vi "init_DAC_do_chans.vi"(10 "Sample Rate":dbl) -> (0 "error out":errorcluster, 2 "Number Chans":dbl, 3 "Refnum out":refnum<k21>)   [LabVIEW 2015]
uses:
  <vilib>/DAQmx/create/channels.llb/DAQmx Create Channel (DO-Digital Output).vi
  <vilib>/DAQmx/configure/timing.llb/DAQmx Timing (Sample Clock).vi
  <resource>/objmgr/daqmx.rc
panel:
  out "Actual Sample Rate":dbl=1000.0 format="%0.2f"
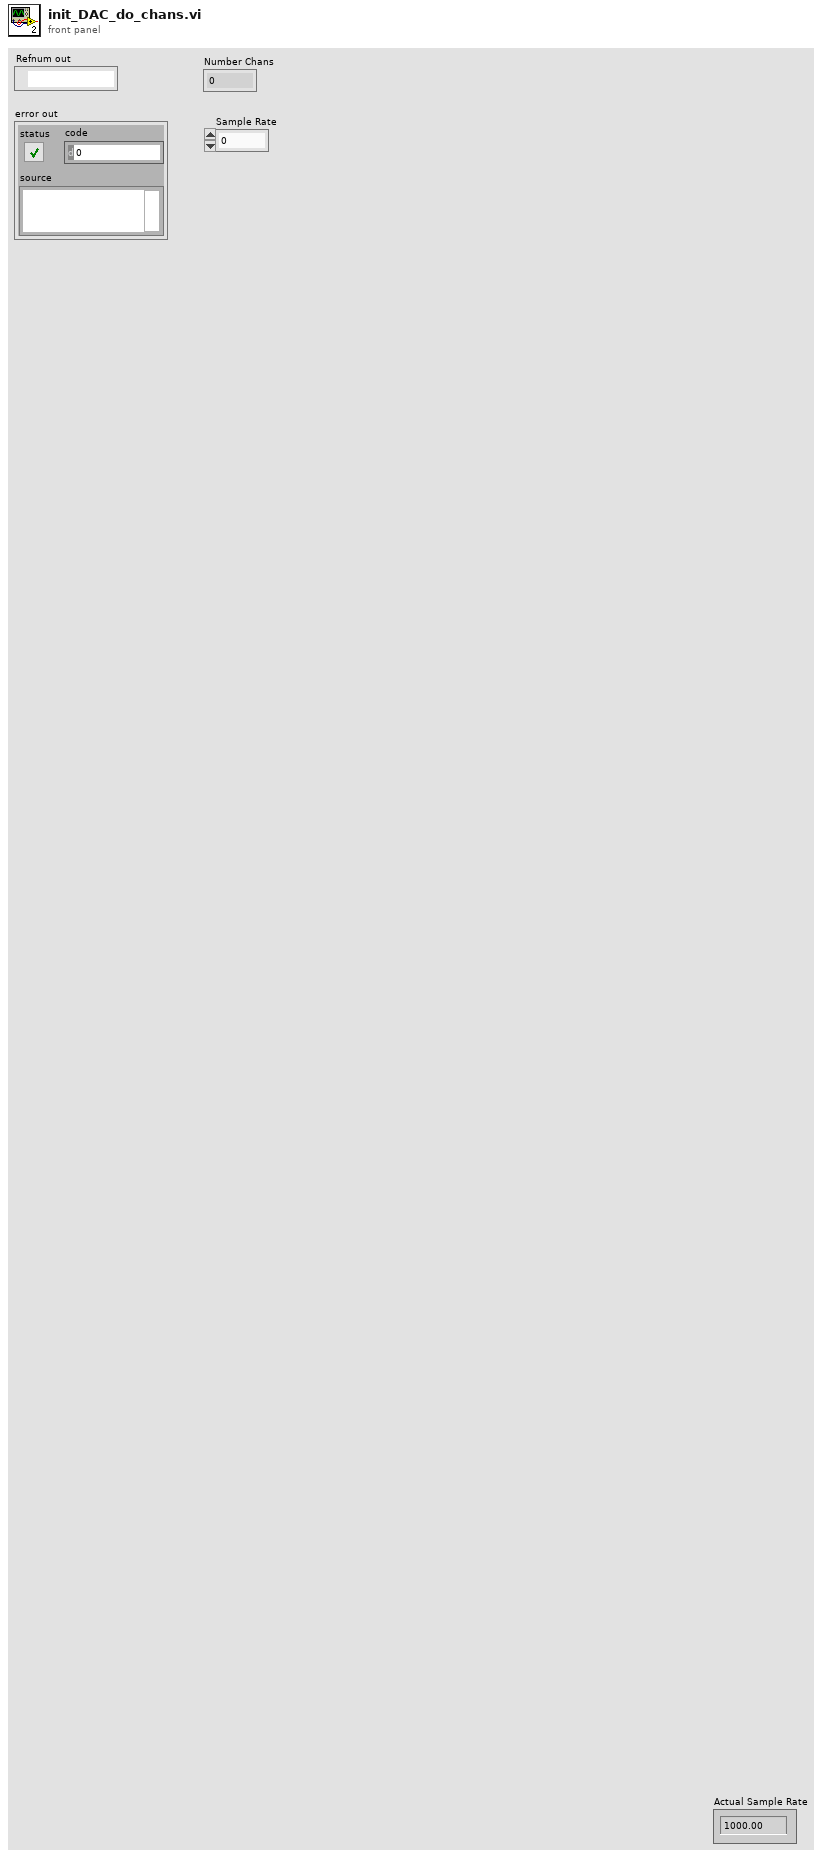
[diagram p1: front panel]
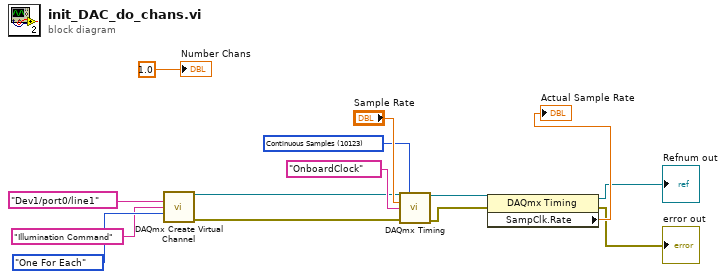
[diagram p0: block diagram]
diagram:
  w3 = 10123 items=["Finite Samples"=10178, "Continuous Samples"=10123] ("sample mode")
  n1 = call-poly <vilib>:"DAQmx Create Virtual Channel.vi"("lines"=tag "Dev1/port0/line1" ("DAQmx Physical Channel"), "name to assign"="Illumination Command", "line grouping"=enum16{"One For Each", "One For All"}."One For Each") -> ("task out"=w2:refnum<k21>, "error out"=w1:errorcluster)  [unwired: 11 in]
  n2 = call-poly <vilib>:"DAQmx Timing.vi"("task/channels in"=w2, "sample mode"=w3, "rate"="Sample Rate", "source"=tag "OnboardClock" ("Sample Clock Source"), "error in"=w1) -> ("task out"=w10:refnum<k21>, "error out"=w9:errorcluster)  [unwired: 9 in]
  n3 = property class="DAQmx Timing"(reference=w10, error in=w9) -> (reference out=→"Refnum out":refnum<k21>, error out=→"error out":errorcluster, "SampClk.Rate"=→"Actual Sample Rate":dbl)
  "Number Chans" <- 1.0 ("Number Chans")
